vi "AI Signal Section.vi"(8 "error in (no error)":errorcluster, 11 "Node Ptr":T1 format="%.0x") -> (0 "error out":errorcluster)   [LabVIEW 2021, in "DAQ Analog InOut System Explorer.lvlib"]
uses:
  DAQ Analog InOut System Explorer.lvlib
  <vilib>/NI VeriStand/Custom Device API/Custom Device API.lvlib
  <vilib>/NI VeriStand/Custom Device API/Custom Device Item Ref.ctl
panel:
  in  "Input Configuration":u16(ring)=10083 items=["RSE"=10083, "NRSE"=10078, "Differential"=10106]
  in  "AI MinV":dbl
  in  "AI MaxV":dbl
  in  "Sample Mode":string="Single Point"
  in  "Specific Header":cluster{"Section Name":string}={"Section Name"="Specific Page Settings"}
  in  "General Header":cluster{"Section Name":string}={"Section Name"="General Page Settings"}
  in  "Description":string
  in  "Name":string
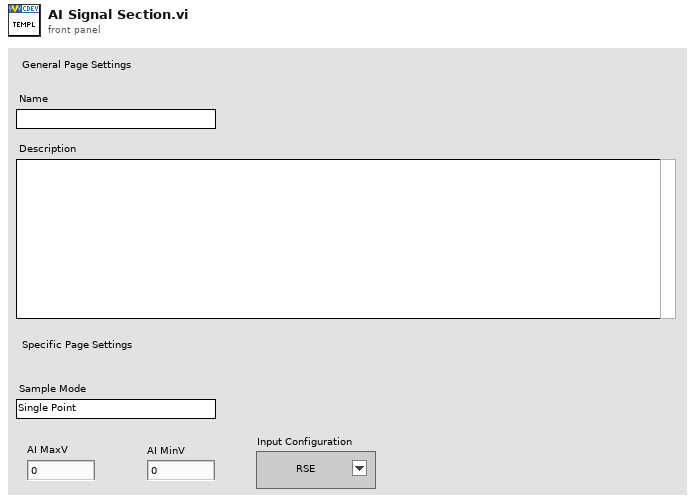
[diagram p1: front panel]
types:
  T1 = typedef "Custom Device API.lvlib/Custom Device Item Ref.ctl" = u64
  T2 = typedef "Custom Device API.lvlib/Custom Device Item Info.ctl" = cluster{"Name":string, "Is Channel":bool, "GUID":string, "Is Waveform":bool}
  T3 = typedef "DAQ Analog InOut System Explorer.lvlib/Input Channel Parameters.ctl" = cluster{"AI MaxV":dbl, "AI MinV":dbl, "Input Configuration":u16}
  T4 = typedef "Custom Device API.lvlib/Custom Device Commands.ctl" = enum16{"Default", "Item renamed", "Shutdown", "Dynamic button pressed"}
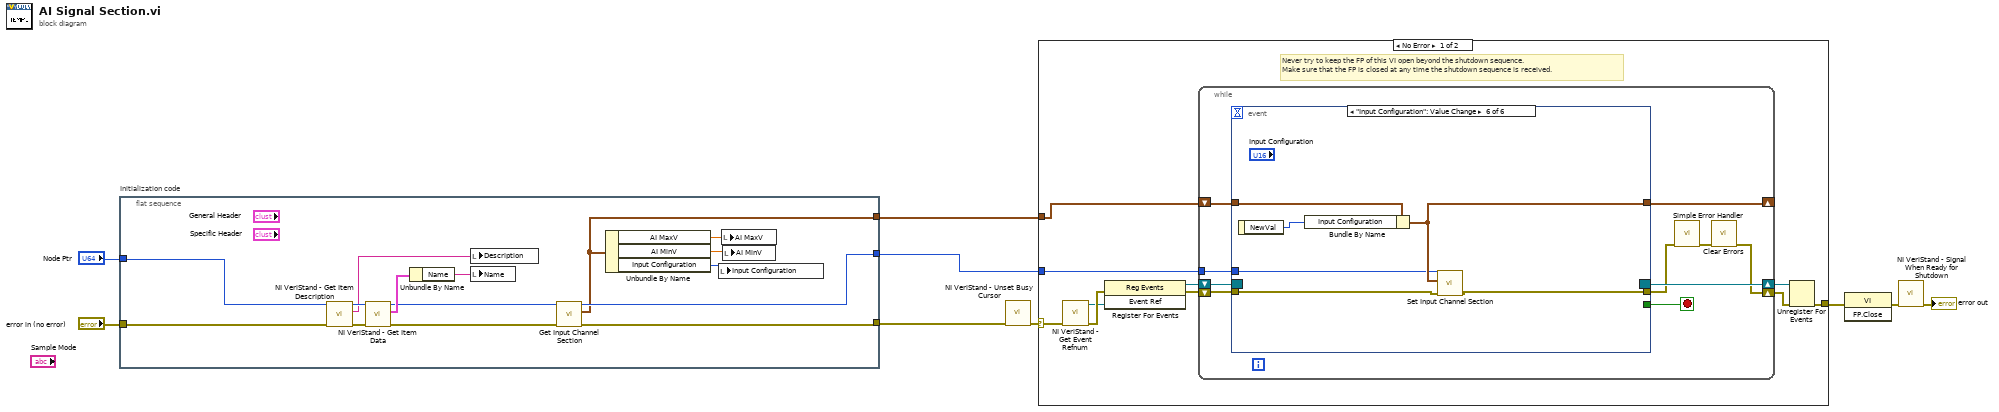
[diagram p0: block diagram]
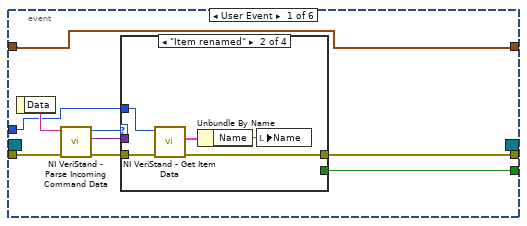
[diagram p2: hidden frame]
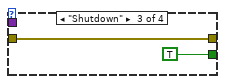
[diagram p4: hidden frame]
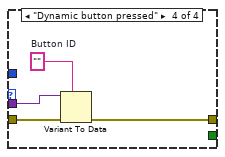
[diagram p5: hidden frame]
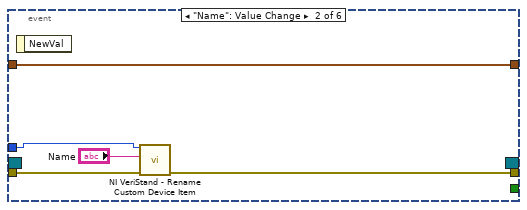
[diagram p6: hidden frame]
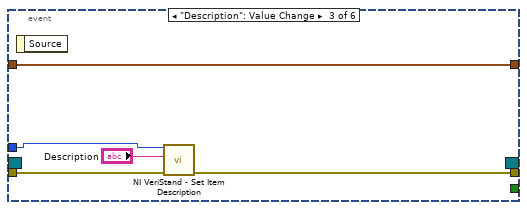
[diagram p7: hidden frame]
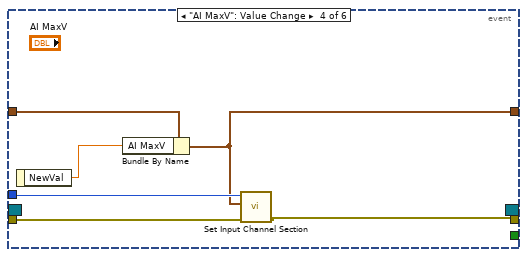
[diagram p8: hidden frame]
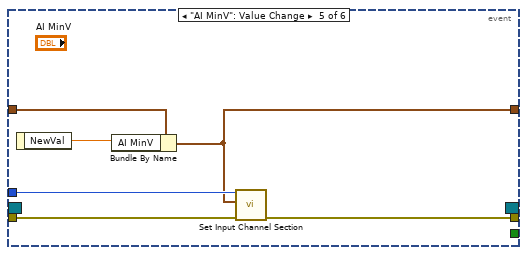
[diagram p9: hidden frame]
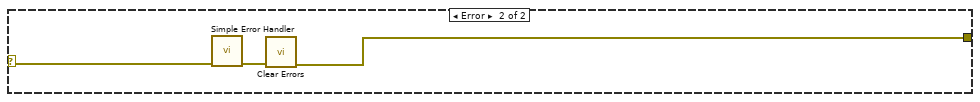
[diagram p10: hidden frame]
diagram:
  n1 = flat-sequence "Initialization code" {
    tunnel: "error in (no error)" -> [w13]
    tunnel: "Node Ptr" -> [w22]
    tunnel: [w16] -> w3
    tunnel: [w15] -> w2
    tunnel: [w14] -> w1
    frame #0 {
      n2 = call <vilib>:"NI VeriStand - Get Item Description.vi"("error in (no error)"=w13, "Item Ref in"=w22) -> ("error out"=w23:errorcluster, "Description"=w20:string, "Item Ref out"=w24:T1)  [unwired: 7 out]
      n3 = call <vilib>:"NI VeriStand - Get Item Data.vi"("error in (no error)"=w23, "Item Ref in"=w24) -> ("error out"=w17:errorcluster, "Item Info"=w19:T2, "Item Ref out"=w18:T1)  [unwired: 7 out]
      n4 = Unbundle By Name(w19) -> ("Name"=w21:string)
      n5 = local write "Description"(w20) -> ()
      n6 = local write "Name"(w21) -> ()
      n7 = call "Get Input Channel Section.vi"("error in (no error)"=w17, "Ref in"=w18) -> ("error out"=w16:errorcluster, "Input Channel Parameters"=w14:T3, "Ref out"=w15:T1)  [unwired: 7 in]
      n8 = Unbundle By Name(w14) -> ("AI MaxV"=w12:dbl, "AI MinV"=w11:dbl, "Input Configuration"=w10:u16)
      n9 = local write "Input Configuration"(w10) -> ()
      n10 = local write "AI MaxV"(w12) -> ()
      n11 = local write "AI MinV"(w11) -> ()
    }
  }
  n12 = call <vilib>:"NI VeriStand - Unset Busy Cursor.vi"("error in (no error)"=w3) -> ("error out"=w5:errorcluster)  [unwired: 10 out]
  n13 = case shown="No Error" w5 {
    selector: w5 -> [w27 w96]
    tunnel: [w31 w94] -> w9
    tunnel: w2 -> [w26 _]
    tunnel: w1 -> [w25 _]
    frame No Error {
      # "Never try to keep the FP of this VI open beyond the shutdown sequence.\nMake sure that the FP is closed at any time the shutdown sequence is received."
      n14 = call <vilib>:"NI VeriStand - Get Event Refnum.vi"("error in (no error)"=w27) -> ("error out"=w34:errorcluster, "Event Ref"=w30:refnum<user-event>)  [unwired: 9 out]
      n15 = register-events(error in=w34, w30) -> (reference out=w28:refnum<event-registration>, error out=w29:errorcluster)  [unwired: 1 in]
      n16 = while {
        shift-right: [w38] -> w32
        shift-left: w29 -> [w43]
        shift-right: [w44] -> w33
        shift-left: w28 -> [w42]
        tunnel: w26 -> [w37]
        shift-right: [w35] -> _
        shift-left: w25 -> [w36]
        stop <- w41 stop-if-true
        n17 = event shown="[5] \"Input Configuration\": Value Change" {
          selector: w42 -> [_ _ _ _ _ _]
          dyn-events: [_ _ _ _ _ _] -> w44
          timeout: _ -> [_ _ _ _ _ _]
          tunnel: w43 -> [w53 w70 w75 w79 w85 w90]
          tunnel: [w49 _ _ _ _ _] -> w41
          tunnel: [w48 w69 w74 w78 w84 w91] -> w40
          tunnel: w37 -> [w45 w67 w72 w77 w83 w88]
          tunnel: w36 -> [w46 w66 w71 w81 w87 w93]
          tunnel: [w46 w66 w71 w76 w82 w89] -> w35
          event User Event {
            n18 = event-data() -> ("Data"=w52:string)  [unwired: 1 out]
            n19 = call <vilib>:"NI VeriStand - Parse Incoming Command Data.vi"("error in (no error)"=w53, "Incoming data"=w52) -> ("error out"=w51:errorcluster, "Outgoing data"=w47:variant, "Action"=w50:T4)  [unwired: 7 out]
            n20 = case shown="\"Item renamed\"" w50 {
              tunnel: w51 -> [w54 w59 w60 w65]
              tunnel: [_ _ TRUE _] -> w49
              tunnel: [w54 w57 w60 w62] -> w48
              tunnel: w47 -> [_ _ _ w64]
              tunnel: w45 -> [_ w55 _ _]
              frame "Default", Default {
              }
              frame "Item renamed" {
                n21 = call <vilib>:"NI VeriStand - Get Item Data.vi"("error in (no error)"=w59, "Item Ref in"=w55) -> ("error out"=w57:errorcluster, "Item Info"=w58:T2)  [unwired: 8 out]
                n22 = Unbundle By Name(w58) -> ("Name"=w56:string)
                n23 = local write "Name"(w56) -> ()
              }
              frame "Shutdown" {
              }
              frame "Dynamic button pressed" {
                w63 = ""  # Button ID
                n24 = Variant To Data(error in=w65, type=w63, Variant=w64) -> (error out=w62:errorcluster)  [unwired: 1 out]
              }
            }
          }
          event "Name": Value Change {
            n25 = event-data() -> ()  [unwired: 2 out]
            n26 = call <vilib>:"NI VeriStand - Rename Custom Device Item.vi"("error in (no error)"=w70, "New Name"="Name", "Item Ref in"=w67) -> ("error out"=w69:errorcluster)  [unwired: 1 in, 7 out]
          }
          event "Description": Value Change {
            n27 = event-data() -> ()  [unwired: 2 out]
            n28 = call <vilib>:"NI VeriStand - Set Item Description.vi"("error in (no error)"=w75, "Description"="Description", "Item Ref in"=w72) -> ("error out"=w74:errorcluster)  [unwired: 8 out]
          }
          event "AI MaxV": Value Change {
            n29 = event-data() -> ("NewVal"=w80:dbl)  [unwired: 1 out]
            n30 = Bundle By Name(cluster=w81, "AI MaxV"=w80) -> (w76:T3)
            n31 = call "Set Input Channel Section.vi"("error in (no error)"=w79, "Input Channel Parameters"=w76, "Ref in"=w77) -> ("error out"=w78:errorcluster)  [unwired: 7 in, 1 out]
          }
          event "AI MinV": Value Change {
            n32 = event-data() -> ("NewVal"=w86:dbl)  [unwired: 1 out]
            n33 = Bundle By Name(cluster=w87, "AI MinV"=w86) -> (w82:T3)
            n34 = call "Set Input Channel Section.vi"("error in (no error)"=w85, "Input Channel Parameters"=w82, "Ref in"=w83) -> ("error out"=w84:errorcluster)  [unwired: 7 in, 1 out]
          }
          event "Input Configuration": Value Change {
            n35 = event-data() -> ("NewVal"=w92:u16)  [unwired: 1 out]
            n36 = Bundle By Name(cluster=w93, "Input Configuration"=w92) -> (w89:T3)
            n37 = call "Set Input Channel Section.vi"("error in (no error)"=w90, "Input Channel Parameters"=w89, "Ref in"=w88) -> ("error out"=w91:errorcluster)  [unwired: 7 in, 1 out]
          }
        }
        n38 = call <vilib>:"Simple Error Handler.vi"("error in (no error)"=w40) -> ("error out"=w39:errorcluster)  [unwired: 1 in, 7 out]
        n39 = call <vilib>:"Clear Errors.vi"("error in (no error)"=w39) -> ("error out"=w38:errorcluster)  [unwired: 1 in, 5 out]
      }
      n40 = Unregister For Events(event registration refnum=w33, error in=w32) -> (error out=w31:errorcluster)
    }
    frame Error {
      n41 = call <vilib>:"Simple Error Handler.vi"("error in (no error)"=w96) -> ("error out"=w95:errorcluster)  [unwired: 1 in, 7 out]
      n42 = call <vilib>:"Clear Errors.vi"("error in (no error)"=w95) -> ("error out"=w94:errorcluster)  [unwired: 1 in, 5 out]
    }
  }
  n43 = invoke class="VI" method="FP.Close"(error in=w9) -> (error out=w8:errorcluster)  [unwired: 2 in, 2 out]
  n44 = call <vilib>:"NI VeriStand - Signal When Ready for Shutdown.vi"("error in (no error)"=w8) -> ("error out"=→"error out":errorcluster)  [unwired: 10 out]
